vi "Send Notifier_Que Kaushik.vi"() -> ()   [LabVIEW 2022 SP3]
panel:
  out "error out":errorcluster
  out "# elements in queue":i32
  out "appended array":i32[](array[numeric])
  in  "stop":bool
  out "Sent Notifier":i8
  in  "Send Que":bool
  in  "Send Notifier":bool
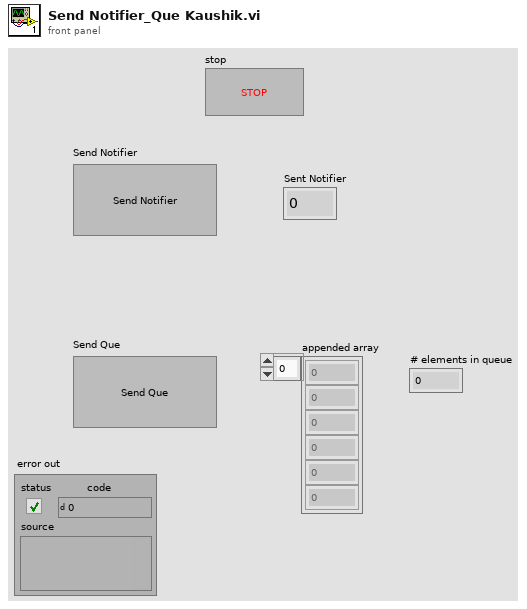
[diagram p1: front panel]
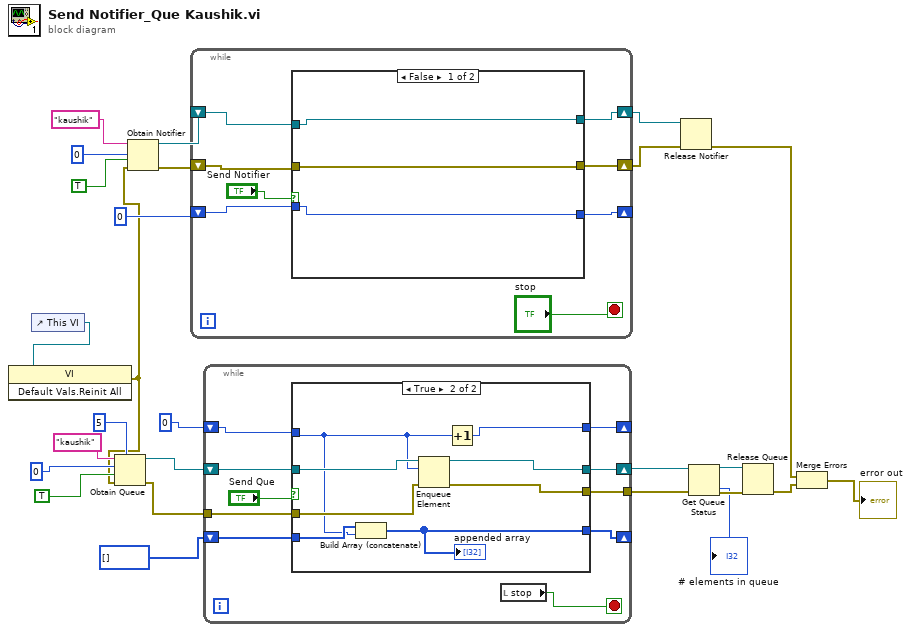
[diagram p0: block diagram]
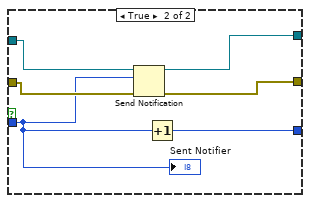
[diagram p3: hidden frame]
diagram:
  n1 = control-ref of="This VI"() -> (w2:refnum<vi>)
  n2 = invoke class="VI" method="Default Vals.Reinit All"(reference=w2) -> (error out=w1:errorcluster)  [unwired: 2 in, 2 out]
  n3 = Obtain Queue(max queue size (-1, unlimited)=5, name (unnamed)="kaushik", element data type=0, create if not found? (T)=TRUE, error in (no error)=w1) -> (queue out=w14:refnum<queue>, error out=w13:errorcluster)  [unwired: 1 out]
  n4 = Obtain Notifier(name (unnamed)="kaushik", notification data type=0, create if not found? (T)=TRUE, error in (no error)=w1) -> (notifier out=w22:refnum<notifier>, error out=w21:errorcluster)  [unwired: 1 out]
  n5 = while {
    shift-right: [w30] -> w20
    shift-left: w22 -> [w31]
    shift-right: [w28] -> w19
    shift-left: w21 -> [w29]
    shift-right: [w32] -> _
    shift-left: 0 -> [w33]
    stop <- "stop" stop-if-true
    n6 = case shown="False" "Send Notifier" {
      tunnel: w33 -> [w35 w38]
      tunnel: [w35 w43] -> w32
      tunnel: w31 -> [w37 w42]
      tunnel: [w37 w41] -> w30
      tunnel: w29 -> [w36 w40]
      tunnel: [w36 w39] -> w28
      frame False {
      }
      frame True {
        n7 = Send Notification(notification=w38, notifier=w42, error in (no error)=w40) -> (notifier out=w41:refnum<notifier>, error out=w39:errorcluster)
        n8 = Increment(x=w38) -> (x+1=w43:i32)
        "Sent Notifier" <- w38
      }
    }
  }
  n9 = while {
    shift-right: [w50] -> _
    shift-left: 0 -> [w51]
    shift-right: [w48] -> w11
    shift-left: w14 -> [w49]
    shift-right: [w44] -> _
    shift-left: i32[] [] -> [w45]
    tunnel: w13 -> [w47]
    tunnel: [w46] -> w10
    stop <- w53 stop-if-true
    n10 = case shown="True" "Send Que" {
      tunnel: w51 -> [w57 w59]
      tunnel: [w57 w65] -> w50
      tunnel: w49 -> [w56 w64]
      tunnel: [w56 w63] -> w48
      tunnel: w47 -> [w55 w62]
      tunnel: [w55 w61] -> w46
      tunnel: w45 -> [w54 w60]
      tunnel: [w54 w58] -> w44
      frame False {
      }
      frame True {
        n11 = Build Array (concatenate)(w60, w59) -> (w58:i32[])
        "appended array" <- w58
        n12 = Enqueue Element(queue=w64, element=w59, error in (no error)=w62) -> (queue out=w63:refnum<queue>, error out=w61:errorcluster)  [unwired: 1 in, 1 out]
        n13 = Increment(x=w59) -> (x+1=w65:i32)
      }
    }
    n14 = local read "stop"() -> (w53:bool)
  }
  n15 = Release Notifier(notifier=w20, error in (no error)=w19) -> (error out=w5:errorcluster)  [unwired: 1 in, 2 out]
  n16 = Get Queue Status(queue=w11, error in (no error)=w10) -> (queue out=w8:refnum<queue>, error out=w9:errorcluster, # elements in queue=→"# elements in queue":i32)  [unwired: 1 in, 5 out]
  n17 = Release Queue(queue=w8, error in (no error)=w9) -> (error out=w6:errorcluster)  [unwired: 1 in, 2 out]
  n18 = Merge Errors(w5, w6) -> (→"error out":errorcluster)
